vi "Restore Configuration.vi"(8 "error in (no error)":errorcluster, 10 "File path":path, 11 "Measure Object in":refnum<class "Log Record.lvclass">) -> (0 "error out":errorcluster, 1 "Section out":string, 2 "File path out":path, 3 "Measure Object out":refnum<class "Log Record.lvclass">)   [LabVIEW 2020, in "Log Record.lvclass"]
uses:
  Log Record.lvclass
  Process Object/Process Object.lvclass
  Log Record.lvclass/Log Record.ctl
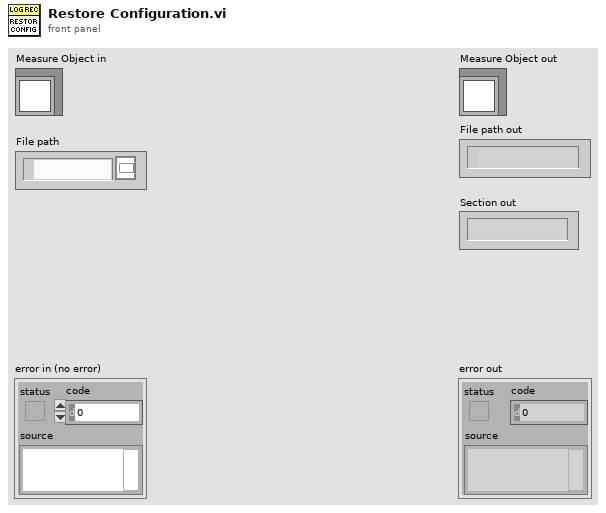
[diagram p1: front panel]
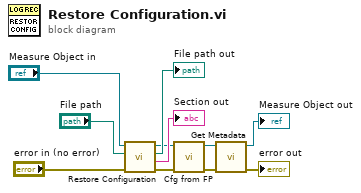
[diagram p0: block diagram]
diagram:
  n1 = call-parent "Restore Configuration.vi"("error in (no error)"="error in (no error)", "File path"="File path", "Measure Object in"="Measure Object in") -> ("error out"=w4:errorcluster, "Section out"=→"Section out":string, "File path out"=→"File path out":path, "Measure Object out"=w3:refnum<class "Log Record.lvclass">)  [unwired: 5 in]
  n2 = call-dynamic "Cfg from FP.vi"("error in (no error)"=w4, "Measure Object in"=w3) -> ("error out"=w1:errorcluster, "Measure Object out"=w2:refnum<class "Log Record.lvclass">)  [unwired: 8 in]
  n3 = call-dynamic "Get Metadata.vi"("error in (no error)"=w1, "Log Record in"=w2) -> ("error out"=→"error out":errorcluster, "Log Record out"=→"Measure Object out":refnum<class "Log Record.lvclass">)  [unwired: 8 in]
